vi "API - Open Connection to DAQ.vi"(8 "error in":errorcluster, 11 "DAQ Address (IP or COM)":string="192.168.1.1") -> (0 "error out":errorcluster, 3 "DAQiFi Device Properties":T1)   [LabVIEW 2021]
doc: "Open a connection to the DAQ and send the initialization commands.\n\nThe DAQ address can be an IP address or a com port eg. \"COM3\"."
uses:
  TypeDefs/TypeDef - Cluster of DAQiFi Device Properties.ctl
  TypeDefs/Enum - Connection Type.ctl
  TCP - Open Connection.vi
  TCP - Send Initialization Command to DAQ.vi
  TCP - Write and Read a Synchronous Message.vi
  TCP - Read LineFeed Terminated String.vi
  USB - Open Connection.vi
  USB - Send Initialization Command to DAQ.vi
  USB - Write and Read a Synchronous Message.vi
  USB - Read LineFeed Terminated String.vi
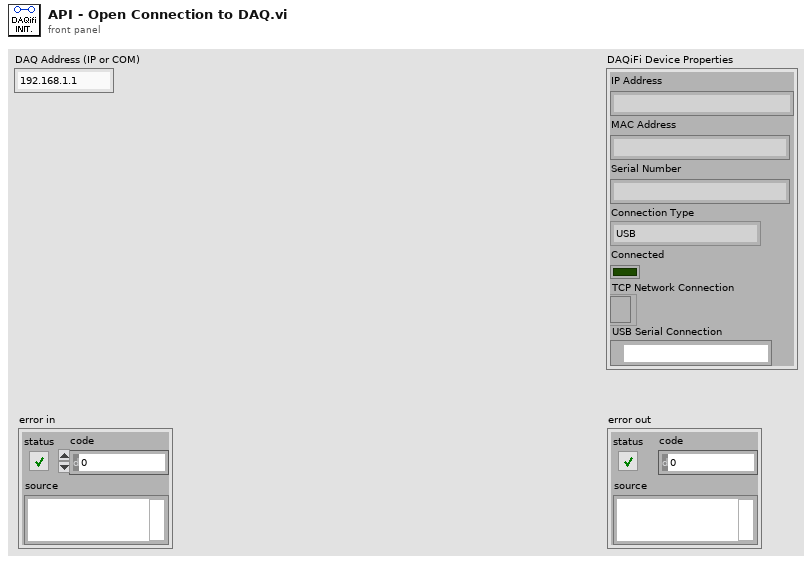
[diagram p1: front panel]
types:
  T1 = typedef "TypeDef - Cluster of DAQiFi Device Properties.ctl" = cluster{"IP Address":string, "MAC Address":string, "Serial Number":string, "Connection Type":T2, "Connected":bool, "TCP Network Connection":refnum<k5>, "USB Serial Connection":refnum<visa-resource-name>}
  T2 = typedef "Enum - Connection Type.ctl" = enum16{"USB", "TCP"}
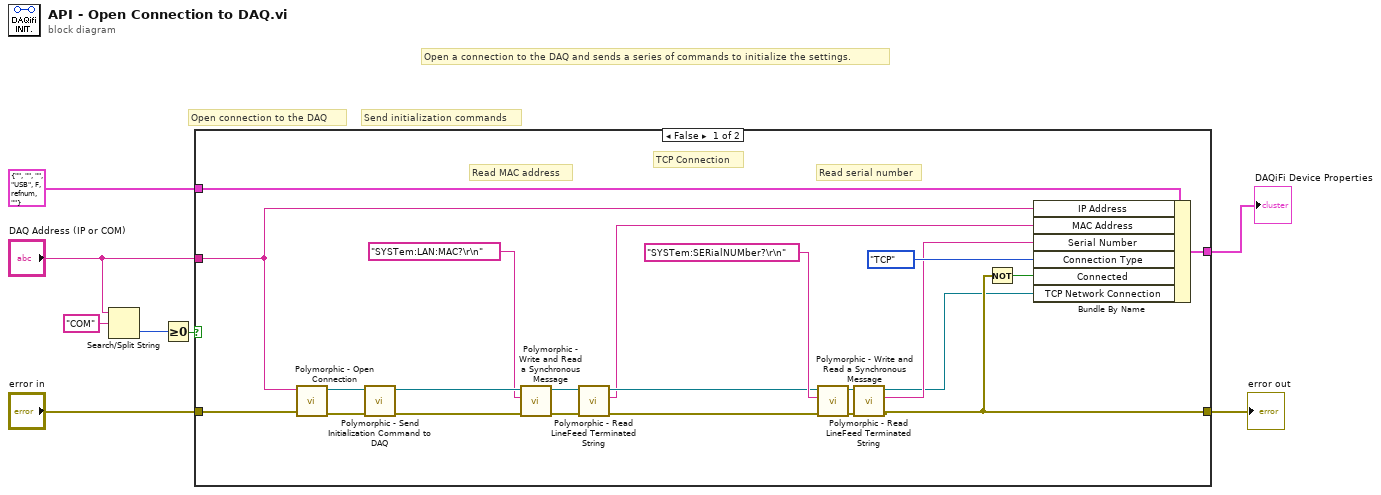
[diagram p0: block diagram]
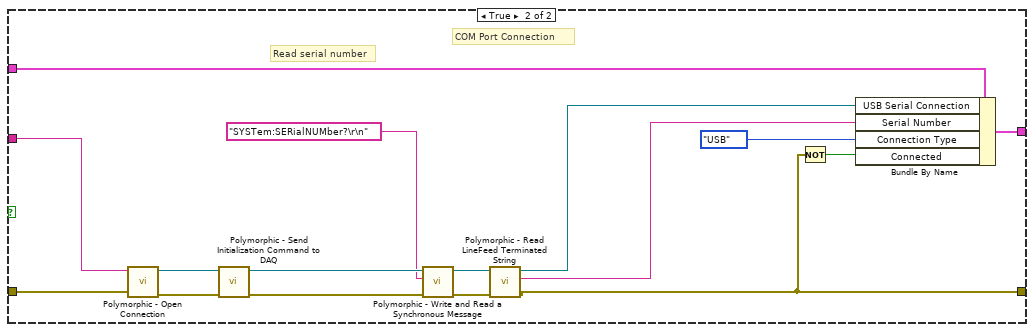
[diagram p2: hidden frame]
diagram:
  # "Open a connection to the DAQ and sends a series of commands to initialize the settings."
  # "Send initialization commands"
  # "Open connection to the DAQ"
  n1 = Search/Split String(string="DAQ Address (IP or COM)", search string/char (-)="COM") -> (offset of match=w5:i32)  [unwired: 1 in, 2 out]
  n2 = Greater Or Equal To 0?(x=w5) -> (x >= 0?=w3:bool)
  n3 = case shown="False" w3 {
    tunnel: [w12 w35] -> w8
    tunnel: "error in" -> [w26 w41]
    tunnel: "DAQ Address (IP or COM)" -> [w25 w42]
    tunnel: T1 {"IP Address"="", "MAC Address"="", "Serial Number"="", "Connection Type"=enum."USB", "Connected"=FALSE, "TCP Network Connection"=refnum, "USB Serial Connection"=""} ("DAQiFi Device - Basic Properties") -> [w30 w46]
    tunnel: [w27 w43] -> w1
    frame False {
      # "TCP Connection"
      # "Read serial number"
      # "Read MAC address"
      n4 = call-poly "Polymorphic - Open Connection.vi"("error in (no error)"=w26, "DAQ IP Address"=w25) -> ("error out"=w20:errorcluster, "TCP Network Connection out"=w24:refnum<k5>)  [unwired: 8 in]
      n5 = call-poly "Polymorphic - Send Initialization Command to DAQ.vi"("error in (no error)"=w20, "TCP Network Connection in"=w24) -> ("error out"=w19:errorcluster, "TCP Network Connection out"=w23:refnum<k5>)  [unwired: 8 in]
      n6 = call-poly "Polymorphic - Write and Read a Synchronous Message.vi"("error in"=w19, "Message to Send"="SYSTem:LAN:MAC?\r\n", "TCP Network Connection in"=w23) -> ("error out"=w18:errorcluster, "TCP Network Connection out"=w22:refnum<k5>)  [unwired: 6 in, 1 out]
      n7 = call-poly "Polymorphic - Read LineFeed Terminated String.vi"("error in"=w18, "TCP Network Connection in"=w22) -> ("error out"=w17:errorcluster, "Received Text"=w11:string, "TCP Network Connection out"=w13:refnum<k5>)  [unwired: 7 in]
      n8 = call-poly "Polymorphic - Write and Read a Synchronous Message.vi"("error in"=w17, "Message to Send"="SYSTem:SERialNUMber?\r\n", "TCP Network Connection in"=w13) -> ("error out"=w16:errorcluster, "TCP Network Connection out"=w15:refnum<k5>)  [unwired: 6 in, 1 out]
      n9 = call-poly "Polymorphic - Read LineFeed Terminated String.vi"("error in"=w16, "TCP Network Connection in"=w15) -> ("error out"=w12:errorcluster, "Received Text"=w10:string, "TCP Network Connection out"=w9:refnum<k5>)  [unwired: 7 in]
      n10 = Not(x=w12) -> (.not. x?=w28:bool)
      n11 = Bundle By Name(cluster=w30, "IP Address"=w25, "MAC Address"=w11, "Serial Number"=w10, "Connection Type"=Enum_-_Connection_Type."TCP", "Connected"=w28, "TCP Network Connection"=w9) -> (w27:T1)
    }
    frame True {
      # "COM Port Connection"
      # "Read serial number"
      n12 = call-poly "Polymorphic - Open Connection.vi"("error in"=w41, "COM Port"=w42) -> ("error out"=w32:errorcluster, "VISA resource name out"=w40:refnum<visa-resource-name>)  [unwired: 8 in]
      n13 = call-poly "Polymorphic - Send Initialization Command to DAQ.vi"("error in"=w32, "VISA resource name in"=w40) -> ("error out"=w33:errorcluster, "VISA resource name out"=w39:refnum<visa-resource-name>)  [unwired: 8 in]
      n14 = call-poly "Polymorphic - Write and Read a Synchronous Message.vi"("error in"=w33, "Message to Send"="SYSTem:SERialNUMber?\r\n", "VISA resource name in"=w39) -> ("error out"=w34:errorcluster, "VISA resource name out"=w38:refnum<visa-resource-name>)  [unwired: 6 in, 1 out]
      n15 = call-poly "Polymorphic - Read LineFeed Terminated String.vi"("error in"=w34, "VISA resource name in"=w38) -> ("error out"=w35:errorcluster, "Received Text"=w36:string, "VISA resource name out"=w37:refnum<visa-resource-name>)  [unwired: 7 in]
      n16 = Not(x=w35) -> (.not. x?=w44:bool)
      n17 = Bundle By Name(cluster=w46, "USB Serial Connection"=w37, "Serial Number"=w36, "Connection Type"=Enum_-_Connection_Type."USB", "Connected"=w44) -> (w43:T1)
    }
  }
  "error out" <- w8
  "DAQiFi Device Properties" <- w1
